vi "Write I2C Bus.vi"(8 "error in (no error)":errorcluster, 10 "I2C Bus":T1=enum."Invalid", 11 "navX - I2C in":refnum<class "navX - I2C.lvclass">) -> (0 "error out":errorcluster, 3 "navX - I2C out":refnum<class "navX - I2C.lvclass">)   [LabVIEW 2015, in "navX Library v3.lvlib" / "navX - I2C.lvclass"]
uses:
  navX - I2C.lvclass
  <vilib>/Rock Robotics/SystemInterfaces/i2clib/i2c_bus.ctl
  navX - I2C.lvclass/navX - I2C.ctl
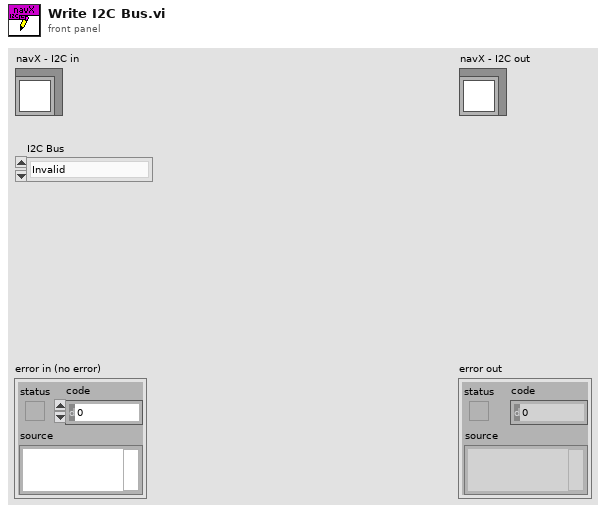
[diagram p1: front panel]
types:
  T1 = typedef "i2c_bus.ctl" = enum16{"I2C On-Board", "I2C MXP", "Invalid"}
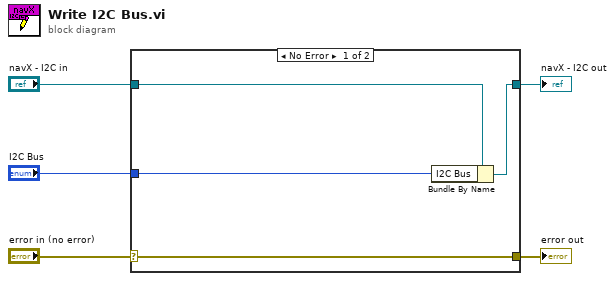
[diagram p0: block diagram]
diagram:
  n1 = case shown="No Error" "error in (no error)" {
    selector: "error in (no error)" -> [w9 w10]
    tunnel: [w9 w10] -> w4
    tunnel: [w7 w11] -> w2
    tunnel: "navX - I2C in" -> [w8 w11]
    tunnel: "I2C Bus" -> [w6 _]
    frame No Error {
      n2 = Bundle By Name(cluster=w8, "I2C Bus"=w6) -> (w7:refnum<class "navX - I2C.lvclass">)
    }
    frame Error {
    }
  }
  "error out" <- w4
  "navX - I2C out" <- w2
